vi "Timeout.vi"(8 "error in (no error)":errorcluster, 11 "Storage Line in":refnum<class "Storage Line.lvclass">) -> (0 "error out":errorcluster, 3 "Storage Line out":refnum<class "Storage Line.lvclass">)   [LabVIEW 2015, in "cRIO-Carbondioxide.lvlib" / "CO2-Actor.lvlib" / "Storage Line.lvclass"]
uses:
  Storage Line.lvclass
panel:
  out "Boolean array":bool[](array[boolean])
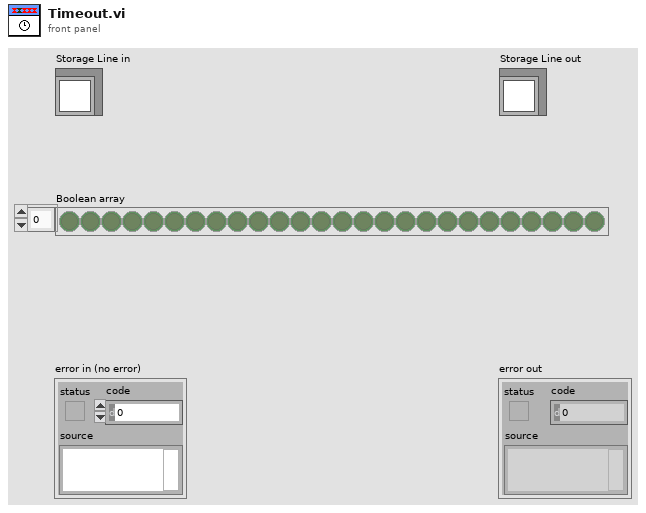
[diagram p1: front panel]
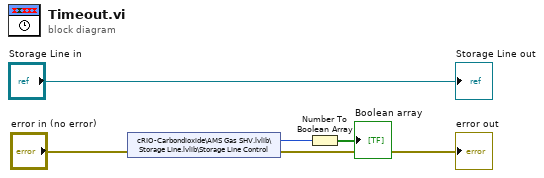
[diagram p0: block diagram]
diagram:
  n1 = shared-variable "cRIO-Carbondioxide\\AMS Gas SHV.lvlib\\Storage Line.lvlib\\Storage Line Control"(error in="error in (no error)") -> (w2:u16, error out=→"error out":errorcluster)
  n2 = Number To Boolean Array(number=w2) -> (Boolean array=→"Boolean array":bool[])
  "Storage Line out" <- "Storage Line in"
